vi "BdcstChannels.vi"(8 "error in (no error)":errorcluster, 9 "Channels":T1, 10 "ModuleID":i32) -> (0 "error out":errorcluster)   [LabVIEW 2014, in "ScopePlugins.lvlib" / "ScopePluginsBase.lvclass"]
uses:
  ScopePluginsBase.lvclass
  TypeDefs/Channels.ctl
  TypeDefs/Channel.ctl
  ScopeModule/Protected/clEventType.ctl
  ScopeModule/ScopeModule.lvlib
  ScopePlugins.lvlib
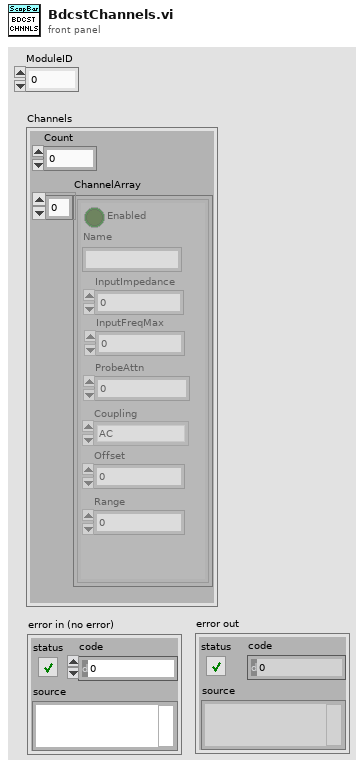
[diagram p1: front panel]
types:
  T1 = typedef "ScopePlugins.lvlib/Channels.ctl" = cluster{"Count":i32, "ChannelArray":T2[]}
  T2 = typedef "ScopePlugins.lvlib/Channel.ctl" = cluster{"Enabled":bool, "Name":string, "InputImpedance":dbl, "InputFreqMax":dbl, "ProbeAttn":dbl, "Coupling":enum16{"AC", "DC", "GND"}, "Offset":dbl, "Range":dbl}
  T3 = typedef "ScopeModule.lvlib/clEventType.ctl" = cluster{"ModuleID":i32, "Data":variant}
  T4 = typedef "ScopeModule.lvlib/clBroadcastEvents.ctl" = cluster{"DidInit":refnum<user-event>, "StatusUpdate":refnum<user-event>, "ErrorReport":refnum<user-event>, "DidStop":refnum<user-event>, "PathToINI":refnum<user-event>, "Handle":refnum<user-event>, "Model":refnum<user-event>, "Channels":refnum<user-event>, "Acquisition":refnum<user-event>, "Trigger":refnum<user-event>}
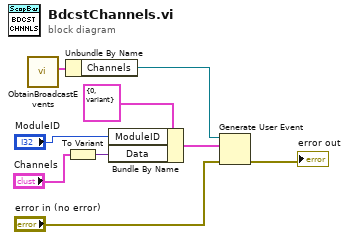
[diagram p0: block diagram]
diagram:
  n1 = call "ObtainBroadcastEvents.vi"() -> ("clBroadcastEvents"=w9:T4)  [unwired: 10 in, 1 out]
  n2 = Unbundle By Name(w9) -> ("Channels"=w8:refnum<user-event>)
  n3 = To Variant(anything="Channels") -> (Variant=w5:variant)
  n4 = Bundle By Name(cluster=T3 {"ModuleID"=0, "Data"=variant} ("clEventType"), "ModuleID"="ModuleID", "Data"=w5) -> (w2:T3)
  n5 = Generate User Event(user event=w8, event data cluster=w2, error in="error in (no error)") -> (error out=→"error out":errorcluster)  [unwired: 1 in, 1 out]
